vi "parse.clz.report.vi"() -> ()   [LabVIEW 2024]
uses:
  <vilib>/Utility/file.llb/Read Delimited Spreadsheet (string).vi
  <userlib>/_OpenG.lib/string/string.llb/openg_string.lvlib
panel:
  out "Array":T1(array[cluster])
  out "header row":string[](array[string])
  in  "error in (no error)":errorcluster
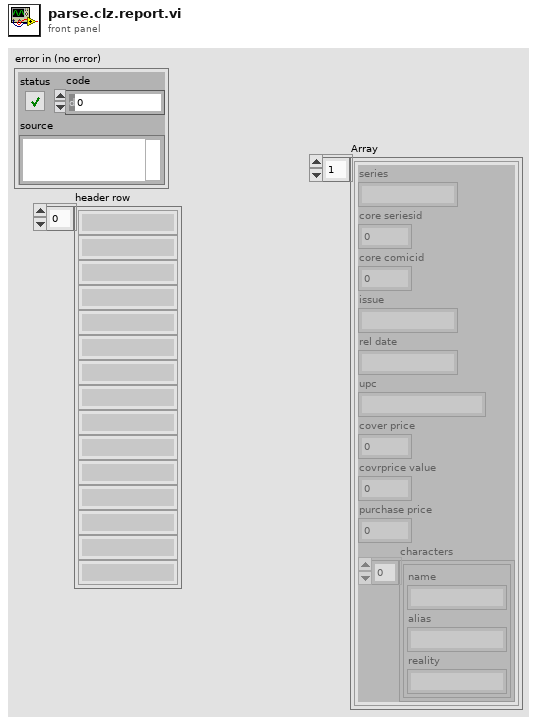
[diagram p1: front panel]
types:
  T1 = cluster{"series":string, "core seriesid":i32, "core comicid":i32, "issue":string, "rel date":string, "upc":string, "cover price":sgl, "covrprice value":sgl, "purchase price":sgl, "characters":cluster{"name":string, "alias":string, "reality":string}[]}[]
  T2 = cluster{"series":string, "core seriesid":i32, "core comicid":i32, "issue":string, "rel date":string, "upc":string, "cover price":sgl, "covrprice value":sgl, "purchase price":sgl, "characters":cluster{"name":string, "alias":string, "reality":string}[]}
  T3 = cluster{"name":string, "alias":string, "reality":string}
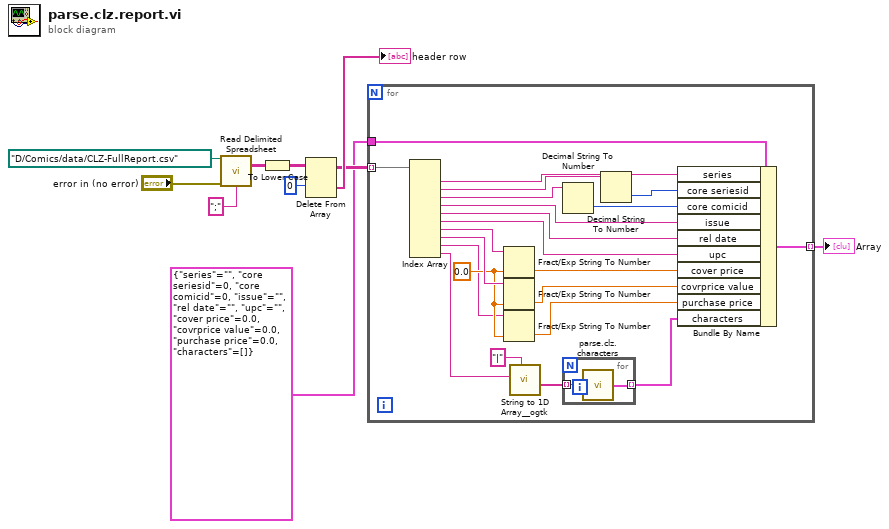
[diagram p0: block diagram]
diagram:
  n1 = call-poly <vilib>:"Read Delimited Spreadsheet.vi"("file path (dialog if empty)"=path "D:/Comics/data/CLZ-FullReport.csv", "error in (no error)"="error in (no error)", "delimiter (\\t)"=";" ("delimiter (\\t)")) -> ("all rows"=w4:string[][])  [unwired: 7 in, 5 out]
  n2 = To Lower Case(string=w4) -> (all lower case string=w3:string[][])
  n3 = Delete From Array(array=w3, index (row)=0) -> (deleted portion=→"header row":string[], array with subset deleted=w5:string[][])  [unwired: 2 in]
  n4 = for {
    tunnel: w5 -> [w32] mode=indexing
    tunnel: T2 {"series"="", "core seriesid"=0, "core comicid"=0, "issue"="", "rel date"="", "upc"="", "cover price"=0.0, "covrprice value"=0.0, "purchase price"=0.0, "characters"=[]} -> [w28]
    tunnel: [w11] -> w1 mode=indexing
    w15 = sgl 0.0
    n5 = Index Array(array=w32) -> (element #1=w27:string, element #2=w26:string, element #3=w24:string, element #4=w22:string, element #5=w21:string, element #6=w20:string, element #7=w18:string, element #8=w16:string, element #9=w14:string, element #10=w29:string)  [unwired: 10 in]
    n6 = Fract/Exp String To Number(string=w18, default (0 dbl)=w15) -> (number=w17:sgl)  [unwired: 2 in, 1 out]
    n7 = Fract/Exp String To Number(string=w16, default (0 dbl)=w15) -> (number=w13:sgl)  [unwired: 2 in, 1 out]
    n8 = Fract/Exp String To Number(string=w14, default (0 dbl)=w15) -> (number=w12:sgl)  [unwired: 2 in, 1 out]
    n9 = call <userlib>:"String to 1D Array__ogtk.vi"("delimiter (Tab)"="|", "string"=w29) -> ("Array of Strings"=w30:string[])  [unwired: 9 in]
    n10 = Decimal String To Number(string=w24) -> (number=w23:i32)  [unwired: 2 in, 1 out]
    n11 = for {
      tunnel: w30 -> [w34] mode=indexing
      tunnel: [w33] -> w19 mode=indexing
      n12 = call "parse.clz.characters.vi"("characters string"=w34) -> ("character"=w33:T3)
    }
    n13 = Decimal String To Number(string=w26) -> (number=w25:i32)  [unwired: 2 in, 1 out]
    n14 = Bundle By Name(cluster=w28, "series"=w27, "core seriesid"=w25, "core comicid"=w23, "issue"=w22, "rel date"=w21, "upc"=w20, "cover price"=w17, "covrprice value"=w13, "purchase price"=w12, "characters"=w19) -> (w11:T2)
  }
  "Array" <- w1
